vi "Module Timeout--constant.vi"() -> (3 "Module Timeout":i32)   [LabVIEW 2021, in "RT Main.lvlib"]
doc: "A module-wide common value to use as the timeout for various synchronization actions.\n_____\nBased on DQMH Dev Tools: Project Template 7.1.2.1547."
uses:
  RT Main.lvlib
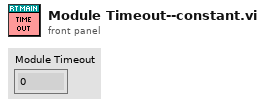
[diagram p1: front panel]
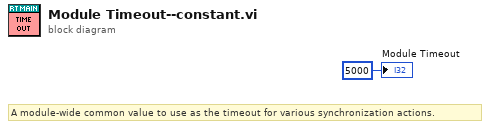
[diagram p0: block diagram]
diagram:
  # "A module-wide common value to use as the timeout for various synchronization actions."
  "Module Timeout" <- 5000 ("Module Timeout")
